vi "ReadMemBlock(U16).vi"(8 "error in (no error)":errorcluster caption="错误输入（无错误）", 11 "标签":string) -> (0 "error out":errorcluster caption="错误输出", 3 "输出值":u16)   [LabVIEW 2012, in "MemBlock.lvlib"]
uses:
  MemBlockTag/MemBlockTagList(U16).vi
  MemBlock/MemBlock(U16).vi
  MemBlock.lvlib
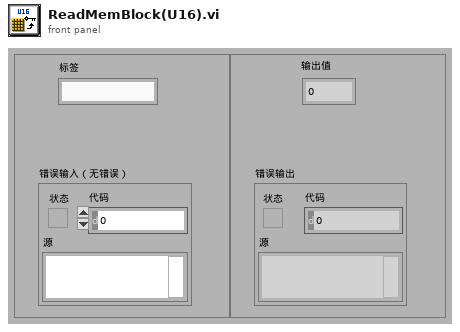
[diagram p1: front panel]
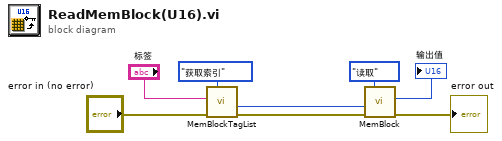
[diagram p0: block diagram]
diagram:
  n1 = call-poly "MemBlockTagList.vi"("方法"=enum16{"初始化", "获取索引"}."获取索引", "error in (no error)"="error in (no error)", "标签"="标签") -> ("error out"=w7:errorcluster, "标签索引"=w6:i32)  [unwired: 6 in, 1 out]
  n2 = call-poly "MemBlock.vi"("方法"=enum16{"初始化", "读取", "读取全部", "写入"}."读取", "error in (no error)"=w7, "索引"=w6) -> ("error out"=→"error out":errorcluster, "输出值"=→"输出值":u16)  [unwired: 6 in, 1 out]
